vi "Synthetic_Jet_Measurement_old.vi"() -> (5 "Plug in titles":string[](array[string]), 7 "Plug in values":string[](array[string]))   [LabVIEW 2012]
uses:
  Controls/SJ_Test_Matrix.ctl
  Controls/Analysis_info_cluster.ctl
  Controls/Inst_type.ctl
  Controls/Instrument_Array.ctl
  Globals/Meas_global.vi
  Globals/Plug_in_data_global.vi
  <vilib>/Analysis/baseanly.llb/Scale 1D.vi
  <vilib>/Analysis/NI_AALBase.lvlib
panel:
  in  "Display Graph?":bool
  out "Normalised Phase Average":cluster{dbl[], "Y=(X-offset)/scale":dbl[]}[](graph)
  in  "Amplitude Steps":i32=9
  in  "Frequency Steps":i32=76
  out "Array":T1[][](array[typedef]) {"Channel Data"."Analysis info cluster"."Sd Error in Variance" format="%.2f"; "Channel Data"."Analysis info cluster"."Skew_u" format="%.2f"; "Channel Data"."Analysis info cluster"."% u'/U" format="%.2f"; "Channel Data"."Analysis info cluster"."Sd Error in Mean" format="%.2f"; "Channel Data"."Analysis info cluster"."Kurt_u" format="%.2f"; "Channel Data"."Analysis info cluster"."u^4" format="%.2f"; "Channel Data"."Analysis info cluster"."u^3" format="%.2f"; "Channel Data"."Analysis info cluster"."U" format="%.2f"; "Channel Data"."Analysis info cluster"."u^2" format="%.2f"}
  out "New Filename":path
  out "Frequency String":string="1200"
  out "Amplitude String":string="3.5000"
  out "Comments":string
  # "You Must have selected the \"Save Data\" option on the \nMeasurement Program for this vi to work correctly"
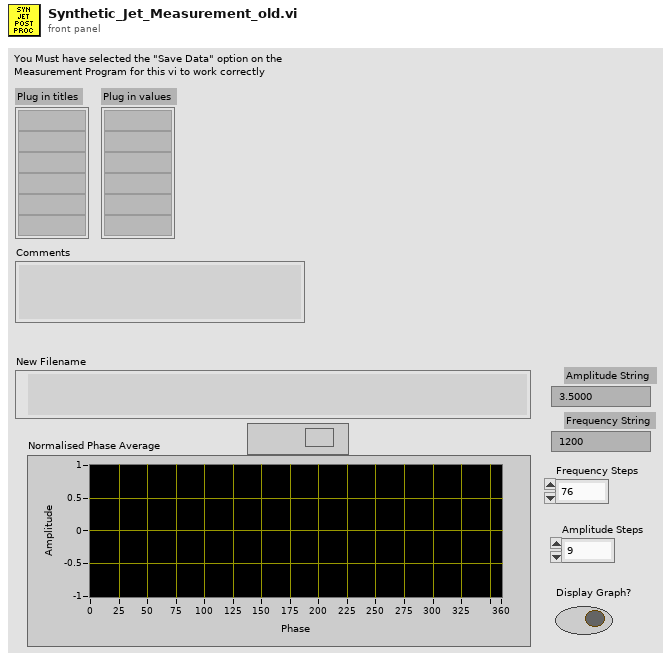
[diagram p1: front panel]
types:
  T1 = typedef "SJ_Test_Matrix.ctl" = cluster{"Channel Data":cluster{"Amplitude (V)":dbl, "Phase Average":dbl[][], "Phase Angle":dbl[], "Frequency (Hz)":dbl, "AS Freq":dbl, "Zero":dbl, "Analysis info cluster":T2, "Radius":dbl[], "||beta||":dbl, "Phi":dbl, "||xd'||":dbl, "xd":dbl[], "||xd||":dbl, "xd'":dbl[], "beta":dbl[]}[]}
  T2 = typedef "Analysis_info_cluster.ctl" = cluster{"Colour":u32, "Inst type":T3, "Inst name":string, "Symbol":string, "Code name":string, "Extra Info":string, "Inst Array":T4, "Extra Titles":string[], "Extra Values":string[], "U":dbl, "u^2":dbl, "u^3":dbl, "u^4":dbl, "Skew_u":dbl, "Kurt_u":dbl, "Sd Error in Mean":dbl, "% u'/U":dbl, "X":dbl, "Y":dbl, "Z":dbl, "Timescale integral to 25%":dbl, "Sd Error in Variance":dbl, "Calib File":path, "Calib Constants":dbl[], "Output Position":bool, "Full Stats":bool, "Av Sampling Rate":dbl, "Av No of Samples":dbl, "Total Meas Time (s)":dbl, "ADAM Ch Name":string}
  T3 = typedef "Inst_type.ctl" = enum16{"Propeller anemometer", "Raw voltage", "Pressure Transducer", "Pitot-static tube", "Preston tube", "Hot wire", "Cross wire 1", "Cross wire 2", "Generic Linear", "Generic Polynomial", "Generic BackPoly", "Fast FID", "Thermocouple", "Cold wire", "Pulsed Wire", "LDA Vel", "LDA Tran time", "LDA Arr time"}
  T4 = typedef "Instrument_Array.ctl" = enum16{"PWA", "LDA", "Analogue"}
  T5 = typedef "Time_Trace_Cluster.ctl" = cluster{"Weighting":dbl[], "Time (s)":dbl[], "Voltage":dbl[], "Eng Values":dbl[]}
  T6 = cluster{"Amplitude (V)":dbl, "Phase Average":dbl[][], "Phase Angle":dbl[], "Frequency (Hz)":dbl, "AS Freq":dbl, "Zero":dbl, "Analysis info cluster":T2, "Radius":dbl[], "||beta||":dbl, "Phi":dbl, "||xd'||":dbl, "xd":dbl[], "||xd||":dbl, "xd'":dbl[], "beta":dbl[]}[]
  T7 = cluster{"Amplitude (V)":dbl, "Phase Average":dbl[][], "Phase Angle":dbl[], "Frequency (Hz)":dbl, "AS Freq":dbl, "Zero":dbl, "Analysis info cluster":T2, "Radius":dbl[], "||beta||":dbl, "Phi":dbl, "||xd'||":dbl, "xd":dbl[], "||xd||":dbl, "xd'":dbl[], "beta":dbl[]}
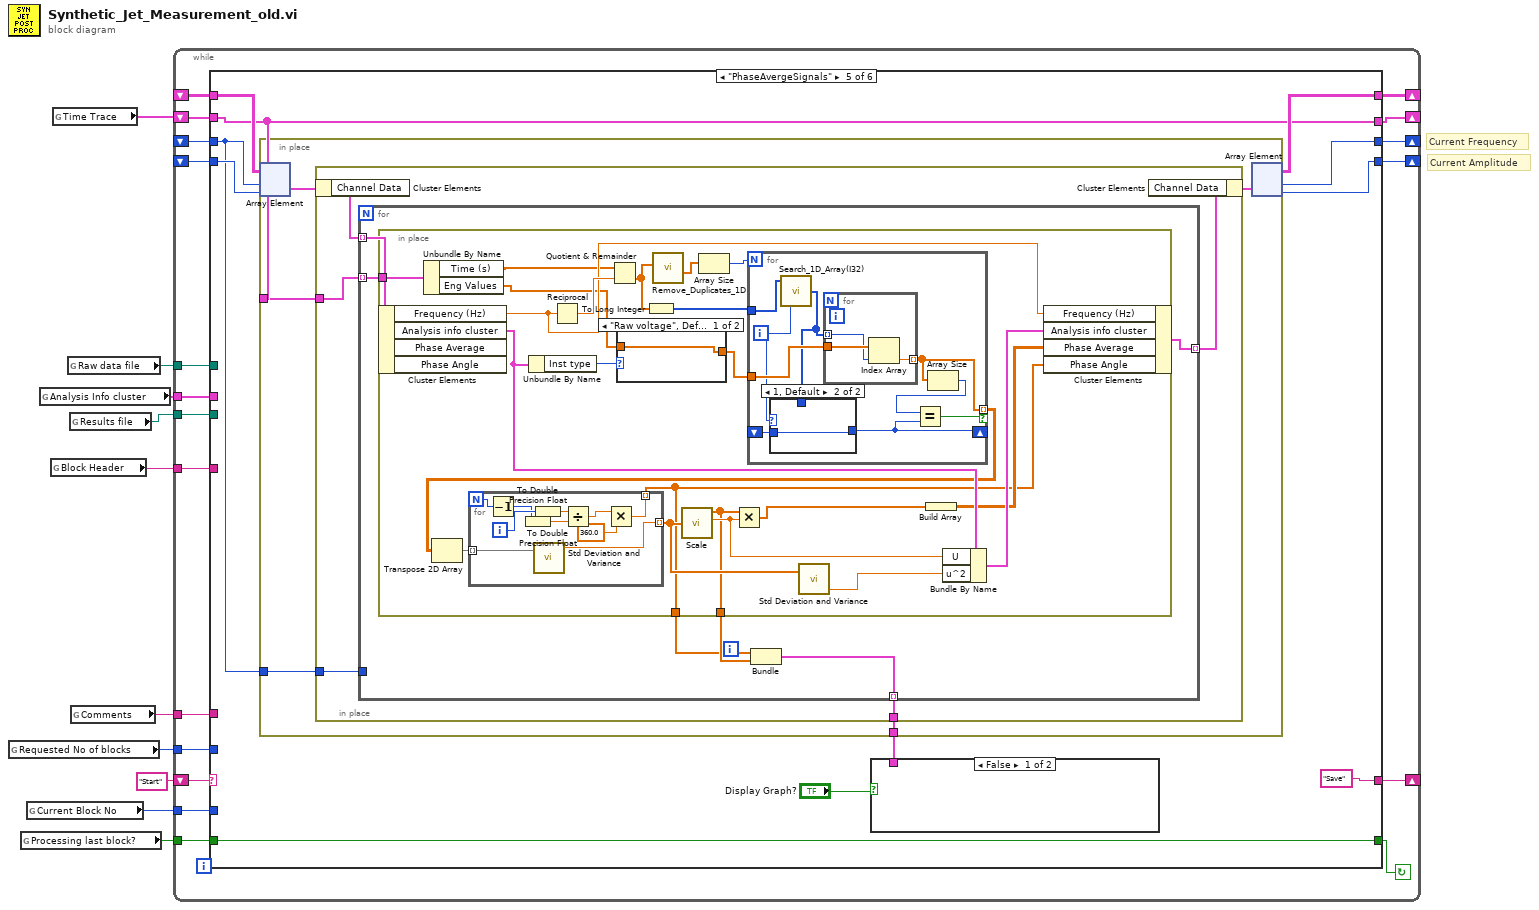
[diagram p0: block diagram]
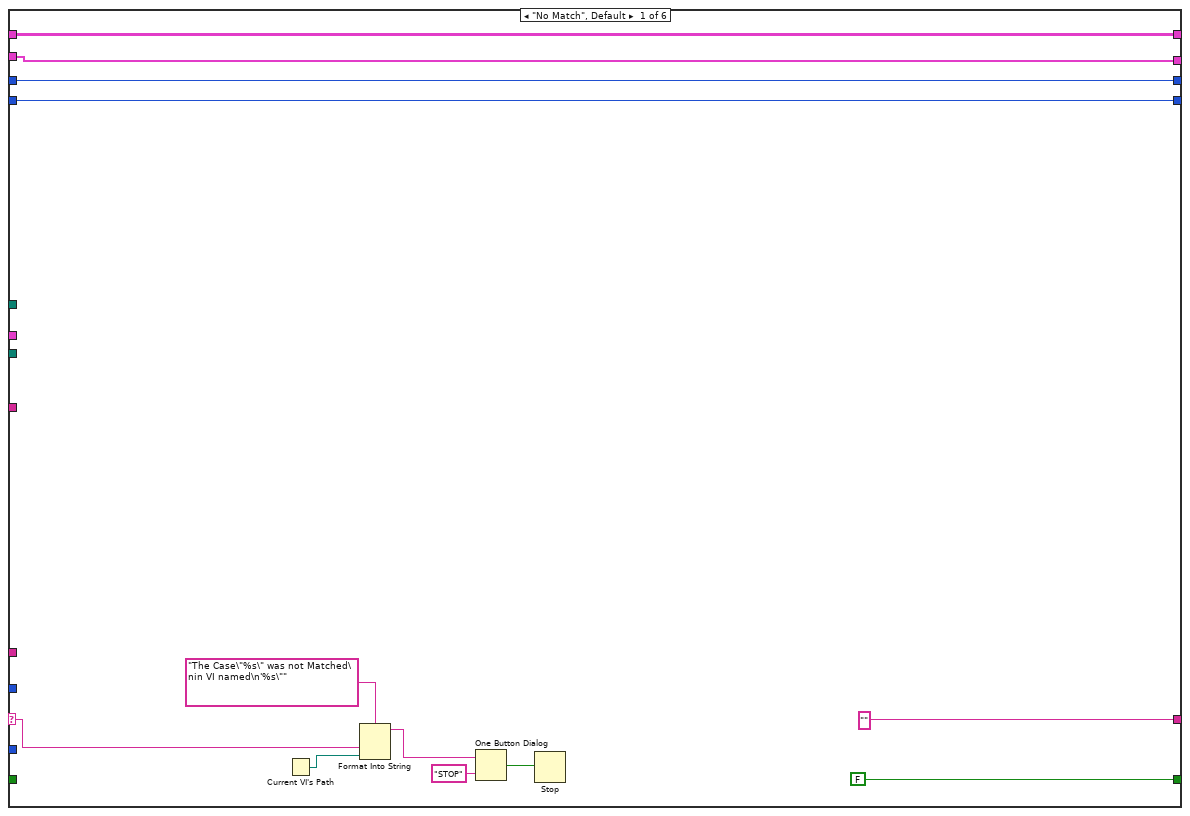
[diagram p2: hidden frame]
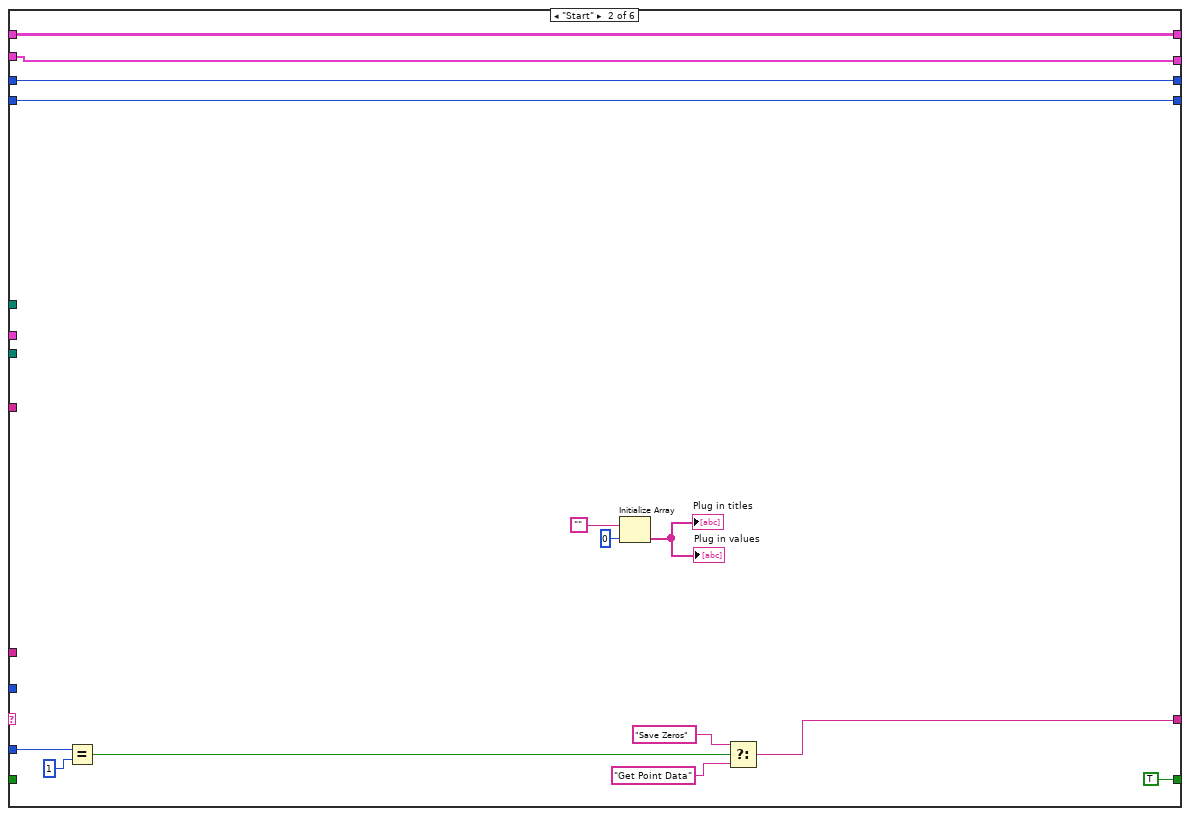
[diagram p3: hidden frame]
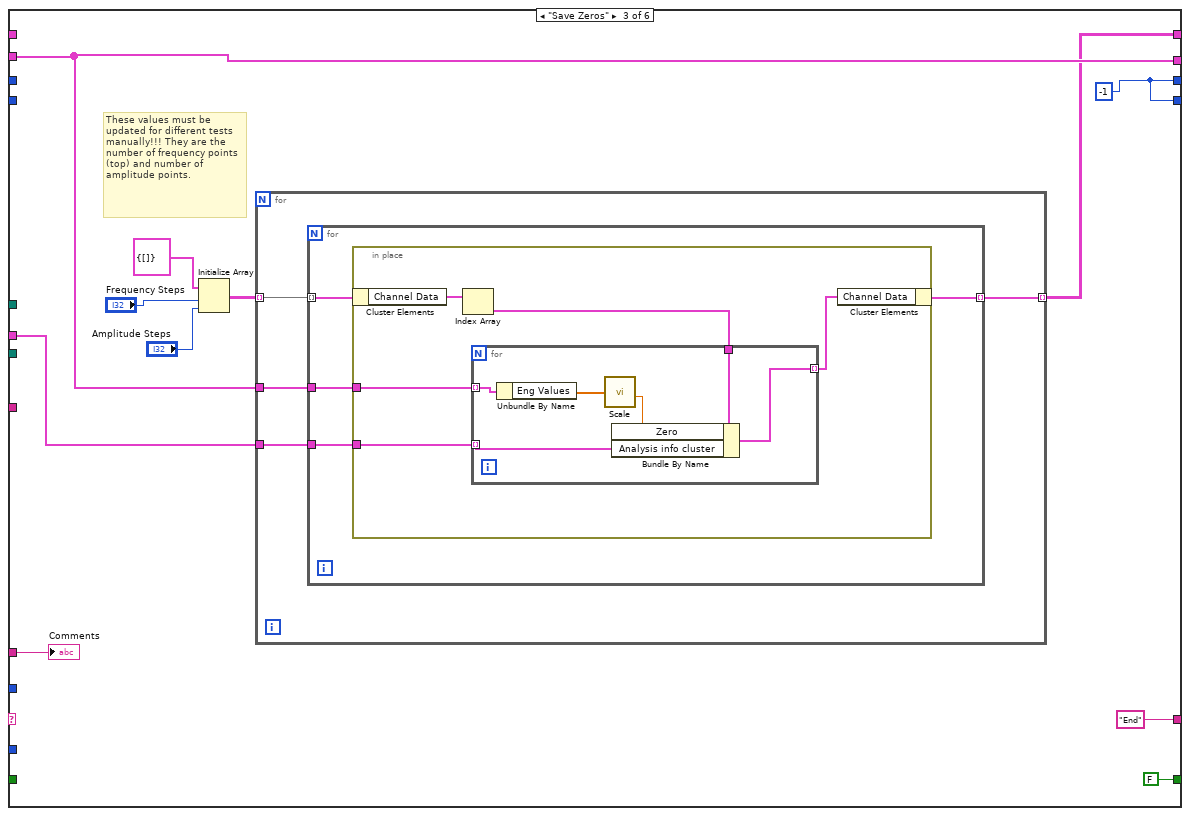
[diagram p4: hidden frame]
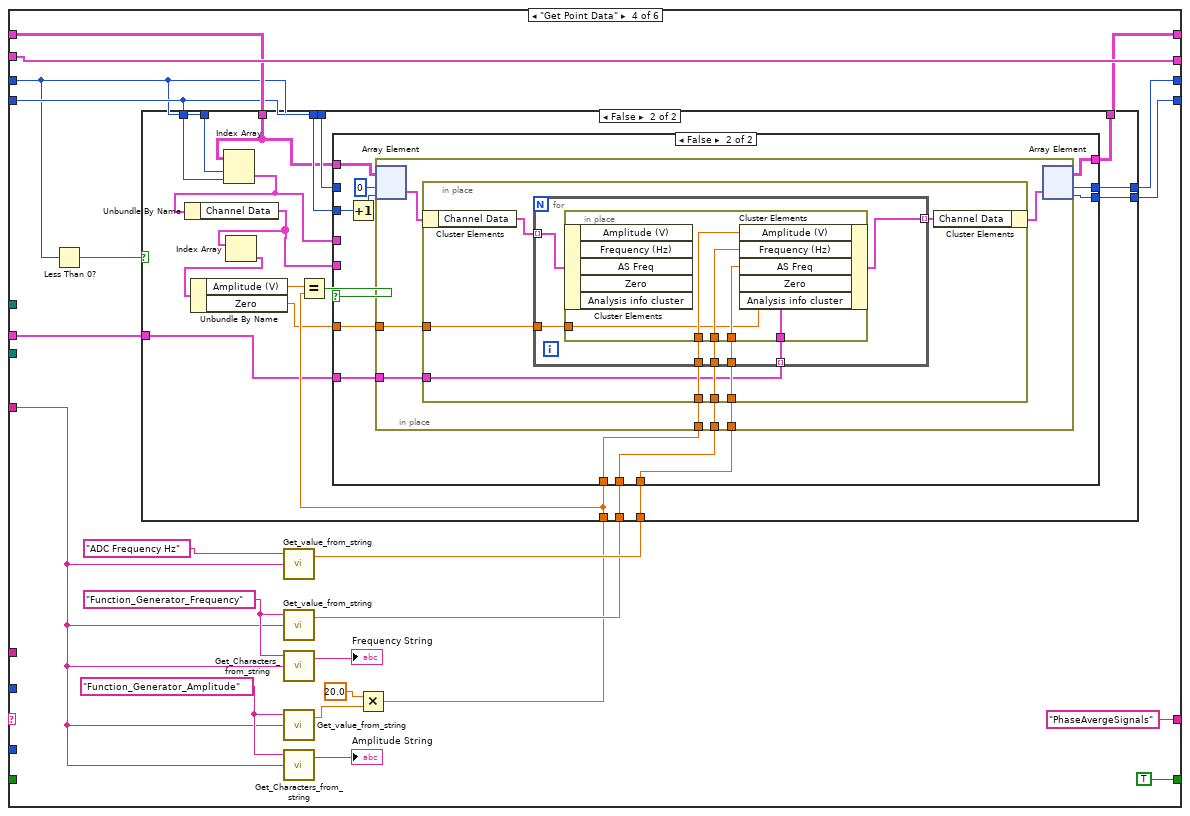
[diagram p5: hidden frame]
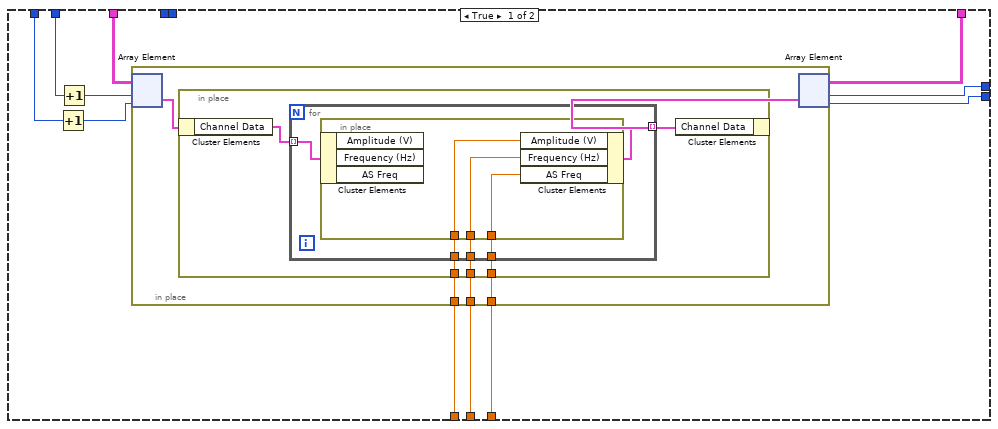
[diagram p6: hidden frame]
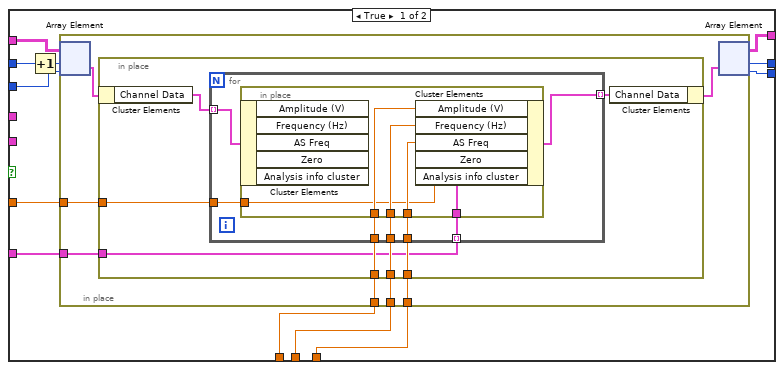
[diagram p7: hidden frame]
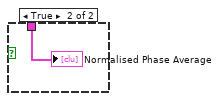
[diagram p8: hidden frame]
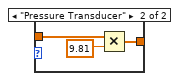
[diagram p9: hidden frame]
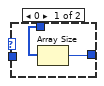
[diagram p10: hidden frame]
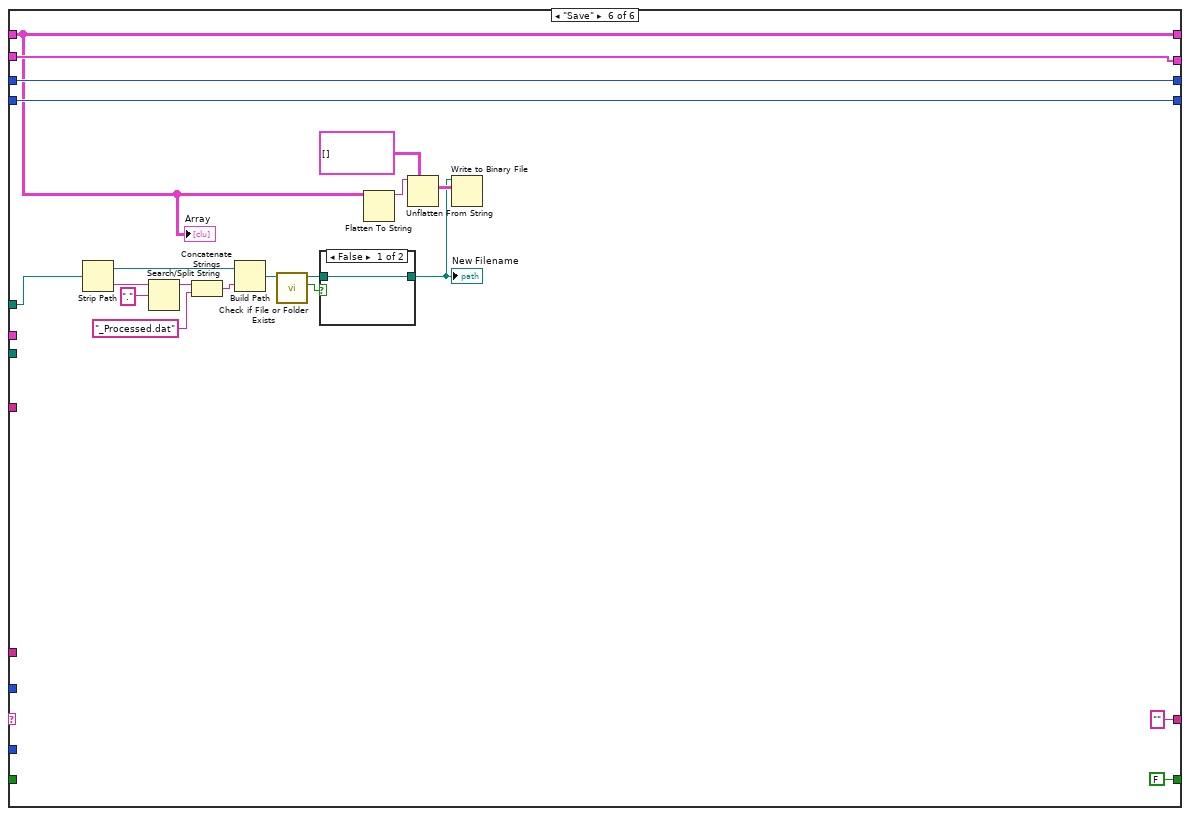
[diagram p11: hidden frame]
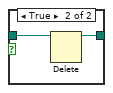
[diagram p12: hidden frame]
diagram:
  # "Current Amplitude"
  # "Current Frequency"
  n1 = global read "Meas_global.vi" "Requested No of blocks"() -> (w6:i32)
  n2 = global read "Meas_global.vi" "Processing last block?"() -> (w5:bool)
  n3 = global read "Meas_global.vi" "Current Block No"() -> (w2:i32)
  n4 = global read "Meas_global.vi" "Analysis Info cluster"() -> (w8:T2[])
  n5 = global read "Plug_in_data_global.vi" "Block Header"() -> (w7:string)
  n6 = global read "Meas_global.vi" "Time Trace"() -> (w3:T5[])
  n7 = global read "Meas_global.vi" "Raw data file"() -> (w9:path)
  n8 = global read "Meas_global.vi" "Results file"() -> (w1:path)
  n9 = global read "Meas_global.vi" "Comments"() -> (w4:string)
  n10 = while {
    shift-left: "Start" -> [w29]
    shift-right: [w22] -> _
    tunnel: w9 -> [w28]
    tunnel: w8 -> [w27]
    tunnel: w7 -> [w25]
    tunnel: w6 -> [w24]
    tunnel: w5 -> [w23]
    shift-right: [w20] -> _
    shift-left: w3 -> [w26]
    tunnel: w4 -> [w19]
    tunnel: w2 -> [w18]
    shift-right: [w16] -> _
    shift-left: _ -> [w17]
    shift-right: [w13] -> _
    shift-left: _ -> [w15]
    shift-right: [w12] -> _
    shift-left: _ -> [w14]
    tunnel: w1 -> [w11]
    stop <- w21 continue-if-true
    n11 = case shown="\"PhaseAvergeSignals\"" w29 {
      selector: w29 -> [w33 _ _ _ _ _]
      tunnel: w28 -> [_ _ _ _ _ w324]
      tunnel: w27 -> [_ _ w63 w89 _ _]
      tunnel: w26 -> [w34 w48 w64 w106 w235 w329]
      tunnel: w25 -> [_ _ _ w96 _ _]
      tunnel: w24 -> [_ _ _ _ _ _]
      tunnel: w23 -> [_ _ _ _ w233 _]
      tunnel: ["" w50 "End" ("t") "PhaseAvergeSignals" ("t") "Save" ("t") "" ("t")] -> w22
      tunnel: [FALSE TRUE FALSE TRUE w233 FALSE ("Processing last block?")] -> w21
      tunnel: [w34 w48 w64 w106 w235 w329] -> w20
      tunnel: w19 -> [_ _ w62 _ _ _]
      tunnel: w18 -> [_ w47 _ _ _ _]
      tunnel: w17 -> [w32 w44 _ w95 w239 w312]
      tunnel: [w32 w44 w56 w94 w238 w312] -> w16
      tunnel: w15 -> [w31 w43 _ w88 w234 w328]
      tunnel: w14 -> [w30 w42 _ w90 w240 w327]
      tunnel: [w31 w43 w61 w86 w237 w328] -> w13
      tunnel: [w30 w42 w61 w87 w236 w327] -> w12
      tunnel: w11 -> [_ _ _ _ _ _]
      frame "No Match", Default {
        n12 = Current VI's Path() -> (path=w37:path)
        n13 = Format Into String(format string="The Case\"%s\" was not Matched\nin VI named\n'%s\"" ("Format String"), w33, w37) -> (resulting string=w40:string)  [unwired: 2 in, 1 out]
        n14 = One Button Dialog(message=w40, button name ("OK")="STOP") -> (true=w38:bool)
        n15 = Stop(stop? (T)=w38) -> ()
      }
      frame "Start" {
        n16 = Equal?(x=w47, y=1) -> (x = y?=w45:bool)
        n17 = Initialize Array("", 0) -> (→"Plug in values" →"Plug in titles":string[])
        n18 = Select(t="Save Zeros", s=w45, f="Get Point Data") -> (s? t:f=w50:string)
      }
      frame "Save Zeros" {
        w61 = -1
        (unwired) "End" ("t")
        (unwired) FALSE ("Processing last block?")
        # "These values must be updated for different tests manually!!! They are the number of frequency points (top) and number of amplitude points."
        n19 = Initialize Array(T1 {"Channel Data"=[]} ("Test Specific Matrix"), "Frequency Steps", "Amplitude Steps") -> (w57:T1[][])
        n20 = for {
          tunnel: w64 -> [w70]
          tunnel: w63 -> [w69]
          tunnel: w57 -> [w68] mode=indexing
          tunnel: [w67] -> w56 mode=indexing
          n21 = for {
            tunnel: w70 -> [w74]
            tunnel: w69 -> [w73]
            tunnel: w68 -> [w72] mode=indexing
            tunnel: [w71] -> w67 mode=indexing
            n22 = in-place {
              in-place-border: w74 -> [w79]
              in-place-border: w73 -> [w78]
              n23 = in-place-cluster #1(w72) -> ("Channel Data"=w77:T6)
              n24 = Index Array(array=w77) -> (element=w76:T7)  [unwired: 1 in]
              n25 = for {
                tunnel: w79 -> [w84] mode=indexing
                tunnel: w78 -> [w82] mode=indexing
                tunnel: w76 -> [w81]
                tunnel: [w80] -> w75 mode=indexing
                n26 = Unbundle By Name(w84) -> ("Eng Values"=w85:dbl[])
                n27 = call-poly <vilib>:"Scale.vi"("X"=w85) -> ("offset"=w83:dbl)  [unwired: 3 out]
                n28 = Bundle By Name(cluster=w81, "Zero"=w83, "Analysis info cluster"=w82) -> (w80:T7)
              }
              n29 = in-place-cluster #1("Channel Data"=w75) -> (w71:T1)
            }
          }
        }
        "Comments" <- w62
      }
      frame "Get Point Data" {
        w100 = "Function_Generator_Amplitude" ("Variable name")
        w101 = "Function_Generator_Frequency" ("Variable name")
        n30 = Less Than 0?(x=w88) -> (x < 0?=w104:bool)
        n31 = call "Get_value_from_string.vi"("Input string"=w96, "Variable name"="ADC Frequency Hz") -> ("Value"=w93:dbl)  [unwired: 1 in, 1 out]
        n32 = call "Get_value_from_string.vi"("Input string"=w96, "Variable name"=w101) -> ("Value"=w92:dbl)  [unwired: 1 in, 1 out]
        n33 = call "Get_Characters_from_string.vi"("Input string"=w96, "Variable name"=w101) -> ("Value"=→"Frequency String":string)  [unwired: 1 in, 1 out]
        n34 = call "Get_value_from_string.vi"("Input string"=w96, "Variable name"=w100) -> ("Value"=w98:dbl)  [unwired: 1 in, 1 out]
        n35 = call "Get_Characters_from_string.vi"("Input string"=w96, "Variable name"=w100) -> ("Value"=→"Amplitude String":string)  [unwired: 1 in, 1 out]
        n36 = Multiply(x=20.0, y=w98) -> (x*y=w91:dbl)
        n37 = case shown="False" w104 {
          tunnel: w88 -> [w118 w150]
          tunnel: w90 -> [w117 w154]
          tunnel: w95 -> [w116 w147]
          tunnel: [w113 w140] -> w94
          tunnel: w93 -> [w112 w146]
          tunnel: w92 -> [w111 w145]
          tunnel: w91 -> [w110 w144]
          tunnel: w88 -> [_ w149]
          tunnel: w90 -> [_ w148]
          tunnel: w89 -> [_ w142]
          tunnel: [w109 w138] -> w86
          tunnel: [w108 w137] -> w87
          frame True {
            n38 = Increment(x=w117) -> (x+1=w114:i32)
            n39 = Increment(x=w118) -> (x+1=w115:i32)
            n40 = in-place {
              in-place-border: w112 -> [w121]
              in-place-border: w111 -> [w120]
              in-place-border: w110 -> [w119]
              n41 = in-place-array #2(w116, w115, w114) -> (w123:T1)
              n42 = in-place {
                in-place-border: w121 -> [w127]
                in-place-border: w120 -> [w126]
                in-place-border: w119 -> [w125]
                n43 = in-place-cluster #3(w123) -> ("Channel Data"=w128:T6)
                n44 = for {
                  tunnel: w128 -> [w133] mode=indexing
                  tunnel: w127 -> [w132]
                  tunnel: w126 -> [w131]
                  tunnel: w125 -> [w130]
                  tunnel: [w129] -> w124 mode=indexing
                  n45 = in-place {
                    in-place-border: w132 -> [w136]
                    in-place-border: w131 -> [w135]
                    in-place-border: w130 -> [w134]
                    n46 = in-place-cluster #4(w133) -> ()  [unwired: 3 out]
                    n47 = in-place-cluster #4("Amplitude (V)"=w134, "Frequency (Hz)"=w135, "AS Freq"=w136) -> (w129:T7)
                  }
                }
                n48 = in-place-cluster #3("Channel Data"=w124) -> (w122:T1)
              }
              n49 = in-place-array #2(w122) -> (w113:T1[][], w109:i32, w108:i32)
            }
          }
          frame False {
            n50 = Index Array(array=w147, index (row)=w150, index (col)=w154) -> (element=w141:T1)
            n51 = Unbundle By Name(w141) -> ("Channel Data"=w143:T6)
            n52 = Index Array(array=w143) -> (element=w153:T7)  [unwired: 1 in]
            n53 = Unbundle By Name(w153) -> ("Amplitude (V)"=w152:dbl, "Zero"=w139:dbl)
            n54 = Equal?(x=w152, y=w144) -> (x = y?=w151:bool)
            n55 = case shown="False" w151 {
              tunnel: w149 -> [w165 _]
              tunnel: w148 -> [w164 w203]
              tunnel: w147 -> [w166 w204]
              tunnel: w146 -> [w162 w201]
              tunnel: w145 -> [w161 w200]
              tunnel: w144 -> [w160 w199]
              tunnel: w143 -> [_ _]
              tunnel: w142 -> [w158 w197]
              tunnel: w141 -> [_ _]
              tunnel: [w163 w202] -> w140
              tunnel: w139 -> [w159 w198]
              tunnel: [w157 w196] -> w138
              tunnel: [w156 w195] -> w137
              frame True {
                n56 = Increment(x=w165) -> (x+1=w155:i32)
                n57 = in-place {
                  in-place-border: w162 -> [w171]
                  in-place-border: w161 -> [w170]
                  in-place-border: w160 -> [w169]
                  in-place-border: w159 -> [w168]
                  in-place-border: w158 -> [w167]
                  n58 = in-place-array #5(w166, w155, w164) -> (w173:T1)
                  n59 = in-place {
                    in-place-border: w171 -> [w179]
                    in-place-border: w170 -> [w178]
                    in-place-border: w169 -> [w177]
                    in-place-border: w168 -> [w175]
                    in-place-border: w167 -> [w174]
                    n60 = in-place-cluster #6(w173) -> ("Channel Data"=w180:T6)
                    n61 = for {
                      tunnel: w180 -> [w187] mode=indexing
                      tunnel: w179 -> [w186]
                      tunnel: w178 -> [w185]
                      tunnel: w177 -> [w184]
                      tunnel: [w183] -> w176 mode=indexing
                      tunnel: w175 -> [w182]
                      tunnel: w174 -> [w181] mode=indexing
                      n62 = in-place {
                        in-place-border: w186 -> [w192]
                        in-place-border: w185 -> [w191]
                        in-place-border: w184 -> [w190]
                        in-place-border: w182 -> [w189]
                        in-place-border: w181 -> [w188]
                        n63 = in-place-cluster #7(w187) -> ()  [unwired: 5 out]
                        n64 = in-place-cluster #7("Amplitude (V)"=w190, "Frequency (Hz)"=w191, "AS Freq"=w192, "Zero"=w189, "Analysis info cluster"=w188) -> (w183:T7)
                      }
                    }
                    n65 = in-place-cluster #6("Channel Data"=w176) -> (w172:T1)
                  }
                  n66 = in-place-array #5(w172) -> (w163:T1[][], w157:i32, w156:i32)
                }
              }
              frame False {
                n67 = Increment(x=w203) -> (x+1=w194:i32)
                n68 = in-place {
                  in-place-border: w201 -> [w209]
                  in-place-border: w200 -> [w208]
                  in-place-border: w199 -> [w207]
                  in-place-border: w198 -> [w206]
                  in-place-border: w197 -> [w205]
                  n69 = in-place-array #8(w204, 0, w194) -> (w211:T1)
                  n70 = in-place {
                    in-place-border: w209 -> [w217]
                    in-place-border: w208 -> [w216]
                    in-place-border: w207 -> [w215]
                    in-place-border: w206 -> [w213]
                    in-place-border: w205 -> [w212]
                    n71 = in-place-cluster #9(w211) -> ("Channel Data"=w218:T6)
                    n72 = for {
                      tunnel: w218 -> [w225] mode=indexing
                      tunnel: w217 -> [w224]
                      tunnel: w216 -> [w223]
                      tunnel: w215 -> [w222]
                      tunnel: [w221] -> w214 mode=indexing
                      tunnel: w213 -> [w220]
                      tunnel: w212 -> [w219] mode=indexing
                      n73 = in-place {
                        in-place-border: w224 -> [w230]
                        in-place-border: w223 -> [w229]
                        in-place-border: w222 -> [w228]
                        in-place-border: w220 -> [w227]
                        in-place-border: w219 -> [w226]
                        n74 = in-place-cluster #10(w225) -> ()  [unwired: 5 out]
                        n75 = in-place-cluster #10("Amplitude (V)"=w228, "Frequency (Hz)"=w229, "AS Freq"=w230, "Zero"=w227, "Analysis info cluster"=w226) -> (w221:T7)
                      }
                    }
                    n76 = in-place-cluster #9("Channel Data"=w214) -> (w210:T1)
                  }
                  n77 = in-place-array #8(w210) -> (w202:T1[][], w196:i32, w195:i32)
                }
              }
            }
          }
        }
      }
      frame "PhaseAvergeSignals" {
        n78 = in-place {
          in-place-border: w235 -> [w245]
          in-place-border: w234 -> [w244]
          in-place-border: [w243] -> w231
          n79 = in-place-array #11(w239, w234, w240) -> (w247:T1)
          n80 = in-place {
            in-place-border: w245 -> [w251]
            in-place-border: w244 -> [w249]
            in-place-border: [w248] -> w243
            n81 = in-place-cluster #12(w247) -> ("Channel Data"=w252:T6)
            n82 = for {
              tunnel: w252 -> [w257] mode=indexing
              tunnel: w251 -> [w258] mode=indexing
              tunnel: [w256] -> w250 mode=indexing
              tunnel: w249 -> [_]
              tunnel: [w253] -> w248 mode=indexing
              n83 = in-place {
                in-place-border: w258 -> [w275]
                in-place-border: [w260] -> w255
                in-place-border: [w259] -> w254
                n84 = in-place-cluster #13(w257) -> ("Frequency (Hz)"=w270:dbl, "Analysis info cluster"=w272:T2)  [unwired: 2 out]
                n85 = Unbundle By Name(w275) -> ("Time (s)"=w265:dbl[], "Eng Values"=w269:dbl[])
                n86 = Unbundle By Name(w272) -> ("Inst type"=w280:T3)
                n87 = Reciprocal(x=w270) -> (1/x=w276:dbl)
                n88 = Quotient & Remainder(x=w265, y=w276) -> (floor(x/y)=w277:dbl[])  [unwired: 1 out]
                n89 = case shown="\"Raw voltage\", Default" w280 {
                  tunnel: w269 -> [w291 w294]
                  tunnel: [w291 w292] -> w279
                  frame "Raw voltage", Default {
                  }
                  frame "Pressure Transducer" {
                    n90 = Multiply(x=w294, y=9.81) -> (x*y=w292:dbl[])
                  }
                }
                n91 = To Long Integer(number=w277) -> (32bit integer=w278:i32[])
                n92 = call "Remove_Duplicates_1D.vi"("Input Array"=w277) -> ("Unique Array"=w274:dbl[])  [unwired: 9 in, 1 out]
                n93 = Array Size(array=w274) -> (size(s)=w273:i32)
                n94 = for {
                  N: w273 -> [_]
                  tunnel: w278 -> [w303]
                  tunnel: w279 -> [w302]
                  tunnel: [w298] -> w267 mode=indexing if=w295
                  shift-right: [w296] -> _
                  shift-left: _ -> [w299]
                  i -> [w301]
                  n95 = call "Search_1D_Array(I32).vi"("Array"=w303, "Element Data"=w301) -> ("Indicies of Elements"=w300:i32[])  [unwired: 6 in, 1 out]
                  n96 = case shown="1, Default" w301 {
                    tunnel: w300 -> [w305 _]
                    tunnel: [w304 w306] -> w296
                    tunnel: w299 -> [_ w306]
                    frame 0 {
                      n97 = Array Size(array=w305) -> (size(s)=w304:i32)
                    }
                    frame 1, Default {
                    }
                  }
                  n98 = for {
                    tunnel: w302 -> [w309]
                    tunnel: w300 -> [w307] mode=indexing
                    tunnel: [w308] -> w298 mode=indexing
                    n99 = Index Array(array=w309, index=w307) -> (element=w308:dbl)
                  }
                  n100 = Array Size(array=w298) -> (size(s)=w297:i32)
                  n101 = Equal?(x=w297, y=w296) -> (x = y?=w295:bool)
                }
                n102 = Transpose 2D Array(2D array=w267) -> (transposed array=w268:dbl[][])
                n103 = for {
                  N -> [w287]
                  tunnel: w268 -> [w290] mode=indexing
                  tunnel: [w289] -> w263 mode=indexing
                  tunnel: [w282] -> w259 mode=indexing
                  i -> [w288]
                  n104 = Decrement(x=w287) -> (x-1=w281:i32)
                  n105 = To Double Precision Float(number=w281) -> (double precision float=w285:dbl)
                  n106 = To Double Precision Float(number=w288) -> (double precision float=w286:dbl)
                  n107 = call <vilib>:"Std Deviation and Variance.vi"("X"=w290) -> ("mean"=w289:dbl)  [unwired: 1 in, 2 out]
                  n108 = Divide(x=w286, y=w285) -> (x/y=w283:dbl)
                  n109 = Multiply(x=w283, y=360.0) -> (x*y=w282:dbl)
                }
                n110 = call-poly <vilib>:"Scale.vi"("X"=w263) -> ("Y=(X-offset)/scale"=w260:dbl[], "scale"=w262:dbl)  [unwired: 2 out]
                n111 = Multiply(x=w260, y=w262) -> (x*y=w261:dbl[])
                n112 = call <vilib>:"Std Deviation and Variance.vi"("X"=w263) -> ("variance"=w264:dbl)  [unwired: 1 in, 2 out]
                n113 = Build Array(w261) -> (w266:dbl[][])
                n114 = Bundle By Name(cluster=w272, "U"=w262, "u^2"=w264) -> (w271:T2)
                n115 = in-place-cluster #13("Frequency (Hz)"=w270, "Analysis info cluster"=w271, "Phase Average"=w266, "Phase Angle"=w259) -> (w256:T7)
              }
              n116 = Bundle(w254, "Y=(X-offset)/scale"=w255) -> (w253:cluster{dbl[], "Y=(X-offset)/scale":dbl[]})  [unwired: 1 in]
            }
            n117 = in-place-cluster #12("Channel Data"=w250) -> (w246:T1)
          }
          n118 = in-place-array #11(w246) -> (w238:T1[][], w237:i32, w236:i32)
        }
        n119 = case shown="False" "Display Graph?" {
          tunnel: w231 -> [_ w242]
          frame False {
          }
          frame True {
            "Normalised Phase Average" <- w242
          }
        }
      }
      frame "Save" {
        n120 = Strip Path(path=w324) -> (stripped path=w321:path, name=w322:string)
        n121 = Search/Split String(string=w322, search string/char (-)=".") -> (substring before match=w320:string)  [unwired: 1 in, 2 out]
        n122 = Concatenate Strings(w320, "_Processed.dat" ("string")) -> (w318:string)
        n123 = Build Path(base path=w321, name or relative path=w318) -> (appended path=w317:path)
        n124 = call <vilib>:"Check if File or Folder Exists.vi"("path"=w317) -> ("file or folder exists?"=w316:bool, "dup path"=w315:path)  [unwired: 8 in, 1 out]
        n125 = case shown="False" w316 {
          tunnel: w315 -> [w330 w332]
          tunnel: [w330 w331] -> w310
          frame False {
          }
          frame True {
            n126 = Delete(path (use dialog)=w332) -> (deleted path=w331:path)  [unwired: 4 in, 2 out]
          }
        }
        "New Filename" <- w310
        n127 = Flatten To String(anything=w312) -> (data string=w314:string)  [unwired: 3 in, 2 out]
        n128 = Unflatten From String(type=T1[][] [], binary string=w314) -> (value=w311:T1[][])  [unwired: 3 in, 2 out]
        n129 = Write to Binary File(file (use dialog)=w310, data=w311) -> ()  [unwired: 4 in, 3 out]
        "Array" <- w312
      }
    }
  }
